vi "DeMux4.vi"(1 "X":bool, 2 "S":bool[](array[boolean])) -> (0 "A":bool[](array[boolean]))   [LabVIEW 2012]
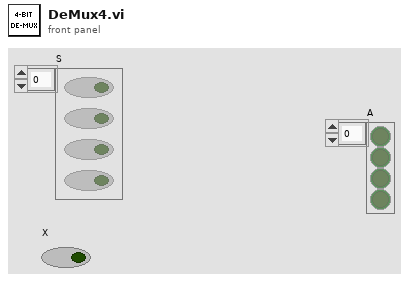
[diagram p1: front panel]
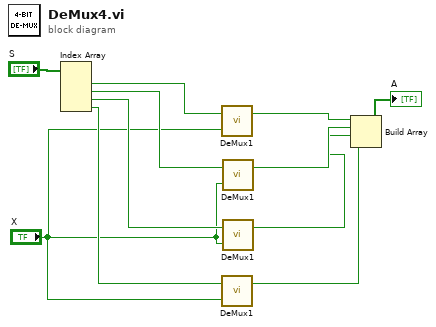
[diagram p0: block diagram]
diagram:
  n1 = Index Array(array="S") -> (element #1=w10:bool, element #2=w9:bool, element #3=w8:bool, element #4=w7:bool)  [unwired: 4 in]
  n2 = call "DeMux1.vi"("X"="X", "S"=w10) -> ("A"=w5:bool)  [unwired: 1 out]
  n3 = call "DeMux1.vi"("X"="X", "S"=w7) -> ("A"=w2:bool)  [unwired: 1 out]
  n4 = call "DeMux1.vi"("X"="X", "S"=w9) -> ("A"=w4:bool)  [unwired: 1 out]
  n5 = call "DeMux1.vi"("X"="X", "S"=w8) -> ("A"=w3:bool)  [unwired: 1 out]
  n6 = Build Array(w5, w4, w3, w2) -> (→"A":bool[])
